vi "LV2Lift.vi"(0 "VerticleMotorControlDevRef":T4={"DeviceStatus"={"status"=FALSE, "code"=0, "source"=""}, "Type"=enum."CAN", "PWM"={"PWM Channel"=enum."PWM 1", "DeadBand"={"Name"="", "maxPositivePwm"=0, "minPositivePwm"=0, "centerPwm"=0, "maxNegativePwm"=0, "minNegativePwm"=0, "angularRange"=0}}, "CAN"={"Device Number"=6, "SetOutput VI Ref"=variant(refnum<vi> refnum), "GetOutput VI Ref"=variant(refnum<vi> refnum), "Enable VI Ref"=variant(refnum<vi> refnum), "Disable VI Ref"=variant(refnum<vi> refnum), "Data"=variant(cluster{"Library":path, "handle":u64, "Control Mode":u16, "UsageFrame":u32, "RefNumName":string, "arbID":u32} {"Library"=path "libCTRE_PhoenixCCI.so", "handle"=53501864, "Control Mode"=0, "UsageFrame"=0, "RefNumName"="LiftElevation", "arbID"=33816582})}, "Invert"=FALSE, "DIO PWM"={"PWM \"Enable\" Channel"=enum."Invalid", "DIOChannel"=enum."Invalid", "PWM Rate"=0.0}}, 9 "Brake DevRef":T1={"DeviceStatus"={"status"=FALSE, "code"=0, "source"=""}, "PWM Channel"=enum."PWM 1", "DeadBand"={"Name"="Servo", "maxPositivePwm"=1770, "minPositivePwm"=1013, "centerPwm"=1007, "maxNegativePwm"=1000, "minNegativePwm"=243, "angularRange"=180}}, 11 "RotationMotorControlDevRef":T4={"DeviceStatus"={"status"=FALSE, "code"=0, "source"=""}, "Type"=enum."CAN", "PWM"={"PWM Channel"=enum."PWM 1", "DeadBand"={"Name"="", "maxPositivePwm"=0, "minPositivePwm"=0, "centerPwm"=0, "maxNegativePwm"=0, "minNegativePwm"=0, "angularRange"=0}}, "CAN"={"Device Number"=7, "SetOutput VI Ref"=variant(refnum<vi> refnum), "GetOutput VI Ref"=variant(refnum<vi> refnum), "Enable VI Ref"=variant(refnum<vi> refnum), "Disable VI Ref"=variant(refnum<vi> refnum), "Data"=variant(cluster{"Library":path, "handle":u64, "Control Mode":u16, "UsageFrame":u32, "RefNumName":string, "arbID":u32} {"Library"=path "libCTRE_PhoenixCCI.so", "handle"=51718392, "Control Mode"=0, "UsageFrame"=0, "RefNumName"="LiftRotation", "arbID"=33816583})}, "Invert"=FALSE, "DIO PWM"={"PWM \"Enable\" Channel"=enum."Invalid", "DIOChannel"=enum."Invalid", "PWM Rate"=0.0}}) -> ()   [LabVIEW 2017]
uses:
  <vilib>/platform/TimedLoop/XDataNode/XDataNode.xnode
  <vilib>/Platform/TimedLoop/XDataNode/nitl_modes.ctl
  <vilib>/Platform/TimedLoop/XDataNode/XDNodeRunTimeDep.lvlib
  <vilib>/Platform/TimedLoop/XDataNode/wakeup.ctl
  <vilib>/Platform/TimedLoop/XDataNode/timing_clust.ctl
  <vilib>/addons/control/pid/NI_PID_pid.lvlib
  <vilib>/addons/control/pid/pid.llb/PID (DBL).vi
  LevelOne/LiftRotLV1Enum.ctl
  LevelOne/VerticalEnum.ctl
  CommandTypes/LiftCommands.ctl
  <vilib>/Rock Robotics/WPI/ThirdParty/Phoenix-LabVIEW/Motor Controller/Controls/CTRE_Phoenix_MotorControl_ControlMode.ctl
  <vilib>/addons/control/pid/pid.llb/PID Output Rate Limiter (DBL).vi
  <vilib>/Rock Robotics/SystemInterfaces/DIO/FPGA_DIOPWMChannel.ctl
  <vilib>/Rock Robotics/WPI/PWM/WPI_PWMDeadband.ctl
  <vilib>/Rock Robotics/WPI/MotorControl/WPI_MotorControlType.ctl
  <vilib>/Rock Robotics/SystemInterfaces/DIO/FPGA_DIOChannel.ctl
  <vilib>/Rock Robotics/WPI/MotorControl/WPI_MotorControlDeviceRef.ctl
  <vilib>/Rock Robotics/WPI/PWM/Servo/WPI_ServoDeviceRef.ctl
panel:
  out "Vertical Lim":cluster{"At Hi":bool, "At Lo":bool}
  out "Vertical Near Lim":cluster{"At Hi near":bool, "At Lo near":bool}
  out "Rotation Arm Current":dbl(graph)
  out "Max Rotation Current":dbl=40.75
  in  "Reset Current Max":bool
  out "Rotation Arm Current":dbl
  in  "Tab Control":T7(tab)=enum."PID"
  in  "Home Desired Rotation":dbl=90.0
  in  "Home Desired Height":dbl=2468.9
  in  "To Scale Low_Desired_Rotation":dbl=54.2584
  in  "To Scale Low_Desired_Height":dbl=16306.2
  in  "To Scale High_Desired_Rotation":dbl=54.2584
  in  "To Scale High_Desired_Height":dbl=26267.9
  in  "To Scale Medium_Desired_Rotation":dbl=54.2584
  in  "To Scale Medium_Desired_Height":dbl=21933.0
  in  "To Switch_Desired_Rotation":dbl=31.0048
  in  "To Switch_Desired_Height":dbl=7119.62
  in  "Ground_Desired_Rotation":dbl
  in  "Ground_Desired_Height":dbl
  in  "Verticle_High_Near_Limit":dbl=4000.0
  in  "Verticle_Low_Limit":dbl=200.0
  in  "Verticle_Low_Near_Limit":dbl=3000.0
  in  "Verticle_Low_Speed_Near_Limit":dbl=0.2
  in  "Verticle_High_Speed_Near_Limit":dbl=0.2
  in  "Verticle_High_Limit":dbl=27000.0
  in  "Vertical coerce":dbl=0.75 format="%#_13g"
  in  "Lift correltion":bool=TRUE
  out "Rotation Tuning Mode?":bool
  in  "Rotation Setpoint":dbl(slide) scale=0.0..100.0
  out "Vertical Tuning Mode?":bool
  in  "Vertical Setpoint":dbl(slide) scale=0.0..30000.0
  out "Vertical Response":cluster{"Value":dbl, "Double":dbl}(graph)={"Value"=7119.62, "Double"=4112.0}
  out "Rotation Response":cluster{"Rotation Setpoint":dbl, "Double":dbl}(graph)={"Rotation Setpoint"=31.0048, "Double"=-8.648384665801359}
  in  "Vertical Min":dbl=-0.9
  in  "Vertical Max":dbl=0.9
  in  "Vertical D Gain":dbl
  in  "Vertical I Gain":dbl
  in  "Vertical P Gain":dbl=0.0001
  in  "Rotation Min":dbl=-1.0
  in  "Rotation Max":dbl=1.0
  in  "Rotation D Gain":dbl=0.002
  in  "Rotation I Gain":dbl=0.01
  in  "Rotation P Gain":dbl=0.03
  in  "rotationalTolerance":dbl=5.0
  in  "Lift_Tolerance":dbl
  in  "Brake Engage Time (s)":dbl
  in  "Brake Servo Engage Angle":dbl
  in  "Brake Servo Disengage Angle":dbl=0.2
  in  "Free_Rotate_Height":dbl=99999.0
  in  "Rotation Feed Forward":dbl(knob)=-0.12604134075051898 scale=1.0..-1.0
  in  "Rot SP Limit":dbl=2000.0 format="%.2f"
  in  "Rotational Manual Power":dbl(knob) scale=0.0..1.0
  in  "Verticle Manual Power":dbl(knob) scale=0.0..1.0
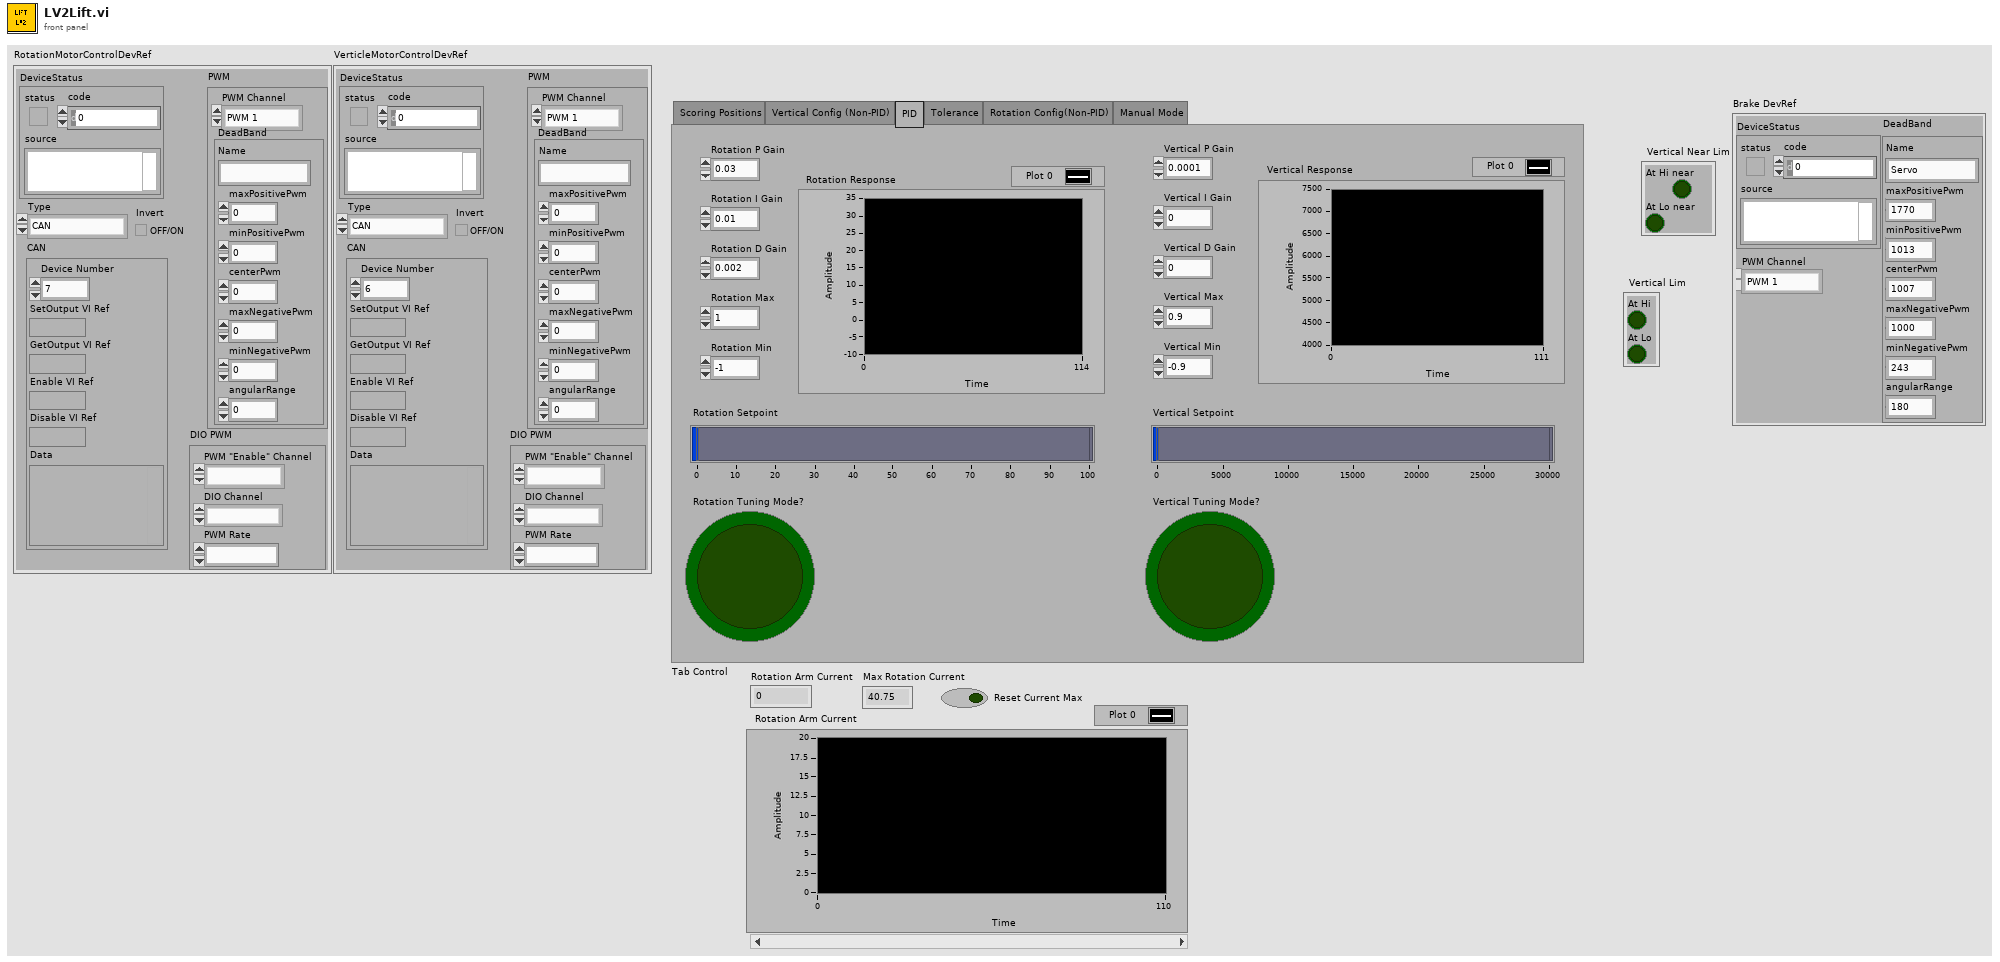
[diagram p1: front panel]
types:
  T1 = typedef "WPI_ServoDeviceRef.ctl" = cluster{"DeviceStatus":errorcluster, "PWM Channel":T2, "DeadBand":T3}
  T2 = typedef "FPGA_DIOPWMChannel.ctl" = enum8{"PWM 0", "PWM 1", "PWM 2", "PWM 3", "PWM 4", "PWM 5", "PWM 6", "PWM 7", "PWM 8", "PWM 9", "PWM MXP 0", "PWM MXP 1", "PWM MXP 2", "PWM MXP 3", "PWM MXP 4", "PWM MXP 5", "PWM MXP 6", "PWM MXP 7", "PWM MXP 8", "PWM MXP 9", "Invalid"}
  T3 = typedef "WPI_PWMDeadband.ctl" = cluster{"Name":string, "maxPositivePwm":i32, "minPositivePwm":i32, "centerPwm":i32, "maxNegativePwm":i32, "minNegativePwm":i32, "angularRange":u16}
  T4 = typedef "WPI_MotorControlDeviceRef.ctl" = cluster{"DeviceStatus":errorcluster, "Type":T5, "PWM":cluster{"PWM Channel":T2, "DeadBand":T3}, "CAN":cluster{"Device Number":u8, "SetOutput VI Ref":variant, "GetOutput VI Ref":variant, "Enable VI Ref":variant, "Disable VI Ref":variant, "Data":variant}, "Invert":bool, "DIO PWM":cluster{"PWM \"Enable\" Channel":T2, "DIOChannel":T6, "PWM Rate":dbl}}
  T5 = typedef "WPI_MotorControlType.ctl" = enum16{"PWM", "CAN", "DIO PWM"}
  T6 = typedef "FPGA_DIOChannel.ctl" = enum8{"DIO 0", "DIO 1", "DIO 2", "DIO 3", "DIO 4", "DIO 5", "DIO 6", "DIO 7", "DIO 8", "DIO 9", "DIO MXP 0", "DIO MXP 1", "DIO MXP 2", "DIO MXP 3", "DIO MXP 4", "DIO MXP 5", "DIO MXP 6", "DIO MXP 7", "DIO MXP 8", "DIO MXP 9", "DIO MXP 10", "DIO MXP 11", "DIO MXP 12", "DIO MXP 13", "DIO MXP 14", "DIO MXP 15", "SPI Port CS1", "SPI Port CS2", "SPI Port CS3", "SPI Port MISO", "SPI Port MOSI", "Invalid"}
  T7 = enum32{"Scoring Positions", "Vertical Config (Non-PID)", "PID", "Tolerance", "Rotation Config(Non-PID)", "Manual Mode"}
  T8 = typedef "LiftCommands.ctl" = enum16{"Do  Nothing", "Manuel", "Home", "Ground", "To Switch", "To Scale Low", "To Scale Medium", "To Scale High"}
  T9 = typedef "XDNodeRunTimeDep.lvlib/timing_clust.ctl" = cluster{"Expected End [f-1]":u64, "Actual End [f-1]":u64, "Finished Late? [f-1]":bool, "Expected End [i-1]":u64, "Actual End [i-1]":u64, "Finished Late? [i-1]":bool, "Expected Start [i]":u64, "Actual Start [i]":u64, "Expected Start [f]":u64, "Actual Start [f]":u64, "Source Name":string, "Structure Name":string, "Period":i64, "Deadline":i64, "Offset":i64, "Start":i64, "Priority":i32, "Timeout":i32, "Mode":T10, "Wakeup Reason":T11, "Error":errorcluster, "Source Type":string, "Secondary Source Type":string, "Global End Time":u64, "Global Start Time":u64, "Frame Duration":u64, "Iteration Duration":u64, "Assigned CPU":i32, "I/O Scan Engine Mode":u32}
  T10 = typedef "XDNodeRunTimeDep.lvlib/nitl_modes.ctl" = enum32{"No Change", "Process missed periods, maintain original phase", "Discard missed periods, maintain original phase", "Process missed periods, ignore original phase", "Discard missed periods, ignore original phase"}
  T11 = typedef "XDNodeRunTimeDep.lvlib/wakeup.ctl" = enum32{"Normal", "Aborted", "Asynchronous wakeup", "Timing source error", "Timed loop error", "Timeout"}
  T12 = typedef "VerticalEnum.ctl" = enum16{"Do Nothing", "Down", "Up"}
  T13 = typedef "LiftRotLV1Enum.ctl" = enum16{"Nothing", "Down", "Up"}
  T14 = cluster{"proportional gain (Kc)":dbl, "integral time (Ti, min)":dbl, "derivative time (Td, min)":dbl}
  T15 = cluster{"Hi Speed near Limit ":dbl, "Lo Speed near Limit":dbl}
  T16 = cluster{"Hi Near Limit ":dbl, "Lo Near Limit":dbl}
  T17 = enum16{"Do  Nothing", "Manuel", "Home", "Ground", "To Switch", "To Scale Low", "To Scale Medium", "To Scale High"}
  T18 = typedef "CTRE_Phoenix_MotorControl_ControlMode.ctl" = u16
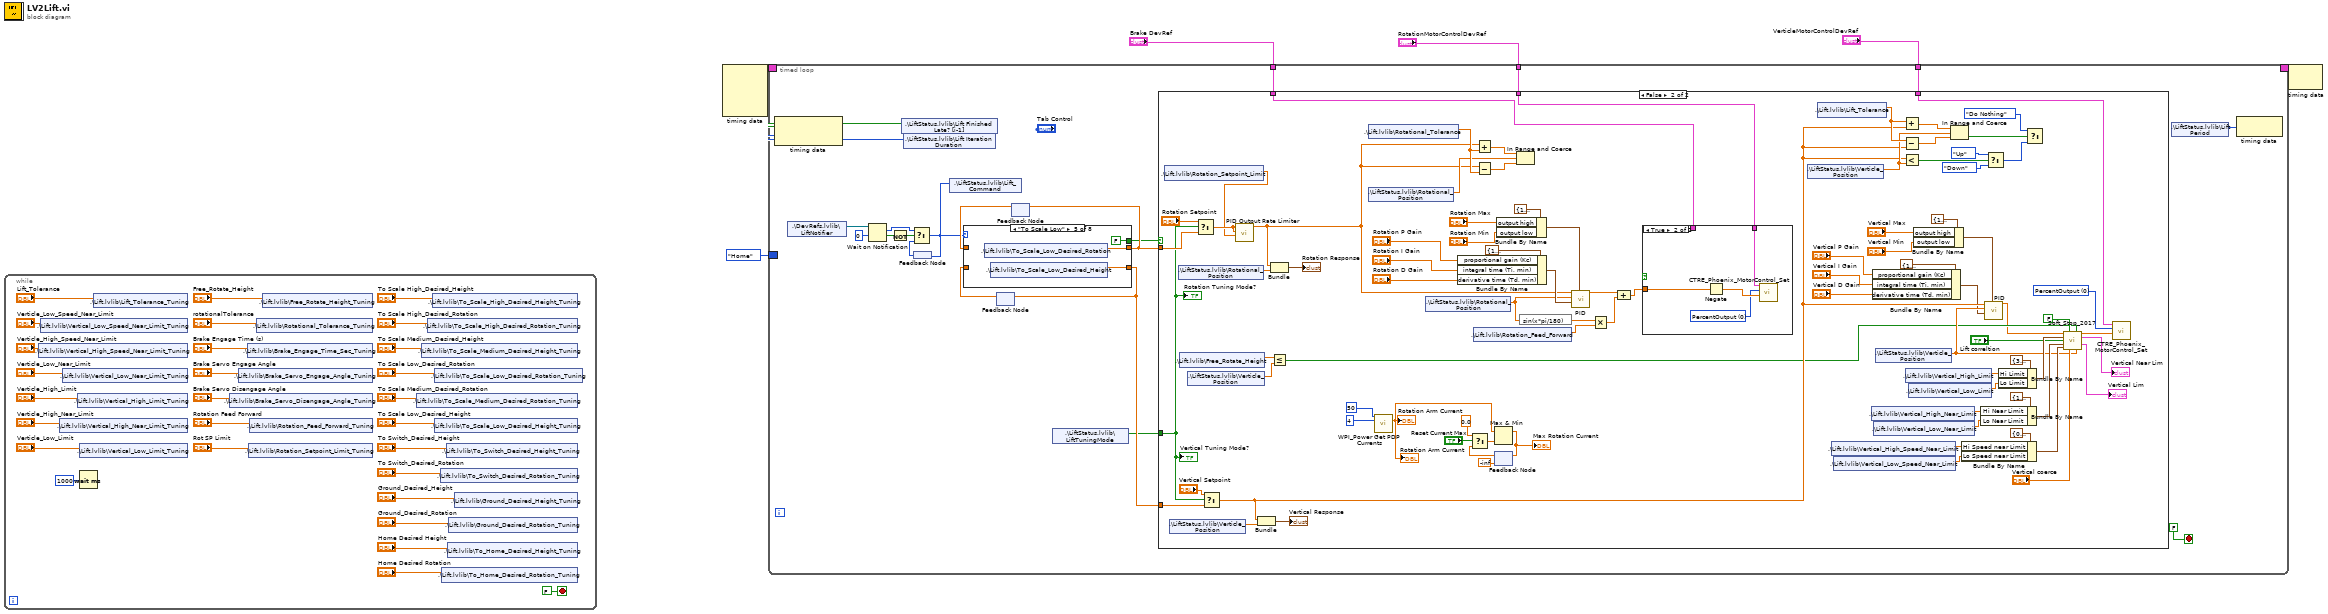
[diagram p0: block diagram]
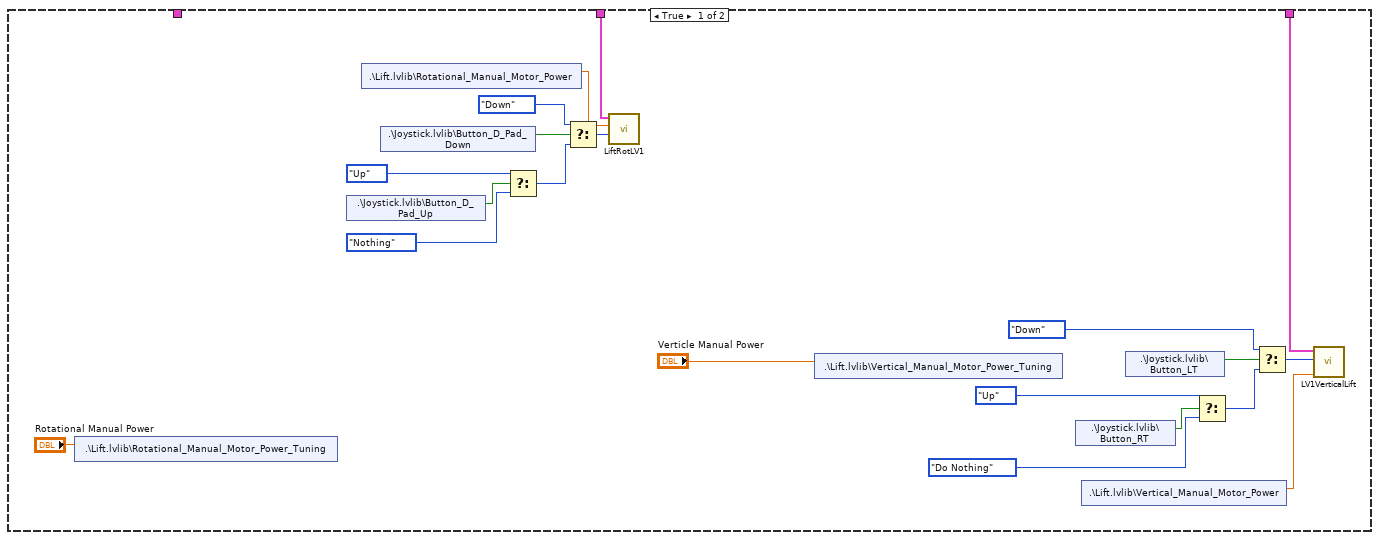
[diagram p2: hidden frame]
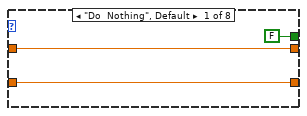
[diagram p4: hidden frame]
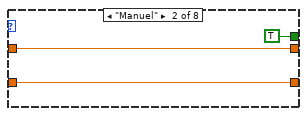
[diagram p5: hidden frame]
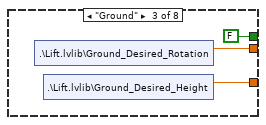
[diagram p6: hidden frame]
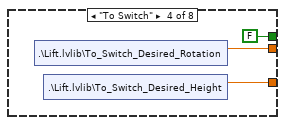
[diagram p7: hidden frame]
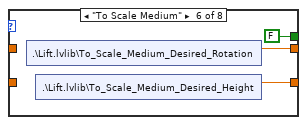
[diagram p8: hidden frame]
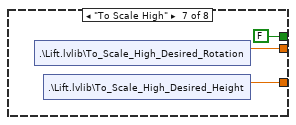
[diagram p9: hidden frame]
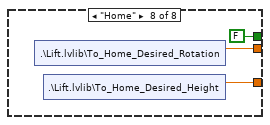
[diagram p10: hidden frame]
diagram:
  n1 = while {
    stop <- FALSE stop-if-true
    n2 = shared-variable ".\\Lift.lvlib\\Vertical_High_Speed_Near_Limit_Tuning"("Verticle_High_Speed_Near_Limit") -> ()  [unwired: 1 in, 1 out]
    n3 = shared-variable ".\\Lift.lvlib\\Vertical_Low_Speed_Near_Limit_Tuning"("Verticle_Low_Speed_Near_Limit") -> ()  [unwired: 1 in, 1 out]
    n4 = shared-variable ".\\Lift.lvlib\\Vertical_High_Near_Limit_Tuning"("Verticle_High_Near_Limit") -> ()  [unwired: 1 in, 1 out]
    n5 = shared-variable ".\\Lift.lvlib\\Vertical_Low_Near_Limit_Tuning"("Verticle_Low_Near_Limit") -> ()  [unwired: 1 in, 1 out]
    n6 = shared-variable ".\\Lift.lvlib\\Vertical_High_Limit_Tuning"("Verticle_High_Limit") -> ()  [unwired: 1 in, 1 out]
    n7 = shared-variable ".\\Lift.lvlib\\Vertical_Low_Limit_Tuning"("Verticle_Low_Limit") -> ()  [unwired: 1 in, 1 out]
    n8 = Wait (ms)(milliseconds to wait=u32 1000) -> ()  [unwired: 1 out]
    n9 = shared-variable ".\\Lift.lvlib\\Lift_Tolerance_Tuning"("Lift_Tolerance") -> ()  [unwired: 1 in, 1 out]
    n10 = shared-variable ".\\Lift.lvlib\\Brake_Servo_Disengage_Angle_Tuning"("Brake Servo Disengage Angle") -> ()  [unwired: 1 in, 1 out]
    n11 = shared-variable ".\\Lift.lvlib\\Brake_Servo_Engage_Angle_Tuning"("Brake Servo Engage Angle") -> ()  [unwired: 1 in, 1 out]
    n12 = shared-variable ".\\Lift.lvlib\\Brake_Engage_Time_Sec_Tuning"("Brake Engage Time (s)") -> ()  [unwired: 1 in, 1 out]
    n13 = shared-variable ".\\Lift.lvlib\\Rotation_Setpoint_Limit_Tuning"("Rot SP Limit") -> ()  [unwired: 1 in, 1 out]
    n14 = shared-variable ".\\Lift.lvlib\\Rotation_Feed_Forward_Tuning"("Rotation Feed Forward") -> ()  [unwired: 1 in, 1 out]
    n15 = shared-variable ".\\Lift.lvlib\\Rotational_Tolerance_Tuning"("rotationalTolerance") -> ()  [unwired: 1 in, 1 out]
    n16 = shared-variable ".\\Lift.lvlib\\Free_Rotate_Height_Tuning"("Free_Rotate_Height") -> ()  [unwired: 1 in, 1 out]
    n17 = shared-variable ".\\Lift.lvlib\\To_Scale_Medium_Desired_Rotation_Tuning"("To Scale Medium_Desired_Rotation") -> ()  [unwired: 1 in, 1 out]
    n18 = shared-variable ".\\Lift.lvlib\\To_Scale_Medium_Desired_Height_Tuning"("To Scale Medium_Desired_Height") -> ()  [unwired: 1 in, 1 out]
    n19 = shared-variable ".\\Lift.lvlib\\To_Scale_High_Desired_Rotation_Tuning"("To Scale High_Desired_Rotation") -> ()  [unwired: 1 in, 1 out]
    n20 = shared-variable ".\\Lift.lvlib\\To_Scale_High_Desired_Height_Tuning"("To Scale High_Desired_Height") -> ()  [unwired: 1 in, 1 out]
    n21 = shared-variable ".\\Lift.lvlib\\To_Scale_Low_Desired_Rotation_Tuning"("To Scale Low_Desired_Rotation") -> ()  [unwired: 1 in, 1 out]
    n22 = shared-variable ".\\Lift.lvlib\\To_Scale_Low_Desired_Height_Tuning"("To Scale Low_Desired_Height") -> ()  [unwired: 1 in, 1 out]
    n23 = shared-variable ".\\Lift.lvlib\\To_Switch_Desired_Rotation_Tuning"("To Switch_Desired_Rotation") -> ()  [unwired: 1 in, 1 out]
    n24 = shared-variable ".\\Lift.lvlib\\To_Home_Desired_Rotation_Tuning"("Home Desired Rotation") -> ()  [unwired: 1 in, 1 out]
    n25 = shared-variable ".\\Lift.lvlib\\To_Switch_Desired_Height_Tuning"("To Switch_Desired_Height") -> ()  [unwired: 1 in, 1 out]
    n26 = shared-variable ".\\Lift.lvlib\\To_Home_Desired_Height_Tuning"("Home Desired Height") -> ()  [unwired: 1 in, 1 out]
    n27 = shared-variable ".\\Lift.lvlib\\Ground_Desired_Rotation_Tuning"("Ground_Desired_Rotation") -> ()  [unwired: 1 in, 1 out]
    n28 = shared-variable ".\\Lift.lvlib\\Ground_Desired_Height_Tuning"("Ground_Desired_Height") -> ()  [unwired: 1 in, 1 out]
  }
  n29 = node-c288() -> (w6:T9)  [unwired: 4 in]
  n30 = timed-loop {
    timing: w6 -> [_]
    timing-out: [_] -> w5
    border: LiftCommands."Home" ("Enum") -> [_]
    tunnel: "VerticleMotorControlDevRef" -> [w43]
    tunnel: "RotationMotorControlDevRef" -> [w42]
    tunnel: "Brake DevRef" -> [w35]
    stop <- FALSE stop-if-true
    n31 = node-c288() -> (w47:bool, w46:i64)  [unwired: 1 in]
    n32 = shared-variable ".\\DevRefs.lvlib\\LiftNotifier"() -> (w54:refnum<notifier>)  [unwired: 1 in, 1 out]
    n33 = Wait on Notification(notifier=w54, timeout in ms (-1)=0) -> (notification=w39:T17, timed out?=w44:bool)  [unwired: 2 in, 2 out]
    n34 = Not(x=w44) -> (.not. x?=w40:bool)
    n35 = shared-variable ".\\LiftStatus.lvlib\\Lift Finished Late? [i-1]"(w47) -> ()  [unwired: 1 in, 1 out]
    n36 = shared-variable ".\\LiftStatus.lvlib\\Lift Iteration Duration"(w46) -> ()  [unwired: 1 in, 1 out]
    n37 = feedback #1() -> (w38:T8)
    n38 = Select(t=w39, s=w40, f=w38) -> (s? t:f=w36:T8)
    n39 = feedback-in #1(w36) -> ()
    n40 = shared-variable ".\\LiftStatus.lvlib\\Lift_Command"(w36) -> ()  [unwired: 1 in, 1 out]
    n41 = feedback #2() -> (w51:dbl)  [unwired: 1 in]
    n42 = feedback #3() -> (w41:dbl)  [unwired: 1 in]
    n43 = case shown="\"To Scale Low\"" w36 {
      tunnel: [w167 w170 w173 w176 w179 w182 w185 w188] -> w50
      tunnel: [w168 w171 w172 w175 w178 w181 w184 w187] -> w52
      tunnel: w51 -> [w168 w171 _ _ _ _ _ _]
      tunnel: w41 -> [w167 w170 _ _ _ _ _ _]
      tunnel: [FALSE TRUE FALSE FALSE FALSE FALSE FALSE FALSE] -> w48
      frame "Do  Nothing", Default {
      }
      frame "Manuel" {
      }
      frame "Ground" {
        n44 = shared-variable ".\\Lift.lvlib\\Ground_Desired_Rotation"() -> (w173:dbl)  [unwired: 1 in, 1 out]
        n45 = shared-variable ".\\Lift.lvlib\\Ground_Desired_Height"() -> (w172:dbl)  [unwired: 1 in, 1 out]
      }
      frame "To Switch" {
        n46 = shared-variable ".\\Lift.lvlib\\To_Switch_Desired_Rotation"() -> (w176:dbl)  [unwired: 1 in, 1 out]
        n47 = shared-variable ".\\Lift.lvlib\\To_Switch_Desired_Height"() -> (w175:dbl)  [unwired: 1 in, 1 out]
      }
      frame "To Scale Low" {
        n48 = shared-variable ".\\Lift.lvlib\\To_Scale_Low_Desired_Rotation"() -> (w179:dbl)  [unwired: 1 in, 1 out]
        n49 = shared-variable ".\\Lift.lvlib\\To_Scale_Low_Desired_Height"() -> (w178:dbl)  [unwired: 1 in, 1 out]
      }
      frame "To Scale Medium" {
        n50 = shared-variable ".\\Lift.lvlib\\To_Scale_Medium_Desired_Rotation"() -> (w182:dbl)  [unwired: 1 in, 1 out]
        n51 = shared-variable ".\\Lift.lvlib\\To_Scale_Medium_Desired_Height"() -> (w181:dbl)  [unwired: 1 in, 1 out]
      }
      frame "To Scale High" {
        n52 = shared-variable ".\\Lift.lvlib\\To_Scale_High_Desired_Rotation"() -> (w185:dbl)  [unwired: 1 in, 1 out]
        n53 = shared-variable ".\\Lift.lvlib\\To_Scale_High_Desired_Height"() -> (w184:dbl)  [unwired: 1 in, 1 out]
      }
      frame "Home" {
        n54 = shared-variable ".\\Lift.lvlib\\To_Home_Desired_Rotation"() -> (w188:dbl)  [unwired: 1 in, 1 out]
        n55 = shared-variable ".\\Lift.lvlib\\To_Home_Desired_Height"() -> (w187:dbl)  [unwired: 1 in, 1 out]
      }
    }
    n56 = feedback-in #2(w52) -> ()
    n57 = feedback-in #3(w50) -> ()
    n58 = shared-variable ".\\LiftStatus.lvlib\\LiftTuningMode"() -> (w37:bool)  [unwired: 1 in, 1 out]
    n59 = case shown="False" w48 {
      tunnel: w52 -> [_ w122]
      tunnel: w50 -> [_ w117]
      tunnel: w43 -> [w59 w82]
      tunnel: w42 -> [w60 w83]
      tunnel: w37 -> [_ w102]
      tunnel: w35 -> [_ w75]
      frame True {
        n60 = shared-variable ".\\Lift.lvlib\\Rotational_Manual_Motor_Power_Tuning"("Rotational Manual Power") -> ()  [unwired: 1 in, 1 out]
        n61 = shared-variable ".\\Joystick.lvlib\\Button_D_Pad_Up"() -> (w66:bool)  [unwired: 1 in, 1 out]
        n62 = shared-variable ".\\Lift.lvlib\\Rotational_Manual_Motor_Power"() -> (w57:dbl)  [unwired: 1 in, 1 out]
        n63 = shared-variable ".\\Joystick.lvlib\\Button_D_Pad_Down"() -> (w65:bool)  [unwired: 1 in, 1 out]
        n64 = Select(t=LiftRotLV1Enum."Up" ("Command"), s=w66, f=LiftRotLV1Enum."Nothing" ("Command")) -> (s? t:f=w74:T13)
        n65 = Select(t=LiftRotLV1Enum."Down" ("Command"), s=w65, f=w74) -> (s? t:f=w72:T13)
        n66 = call "LiftRotLV1.vi"("Command"=w72, "Motor Power"=w57, "PhoenixMotorControlDevRef"=w60) -> ()  [unwired: 9 in]
        n67 = shared-variable ".\\Lift.lvlib\\Vertical_Manual_Motor_Power_Tuning"("Verticle Manual Power") -> ()  [unwired: 1 in, 1 out]
        n68 = shared-variable ".\\Joystick.lvlib\\Button_RT"() -> (w67:bool)  [unwired: 1 in, 1 out]
        n69 = shared-variable ".\\Lift.lvlib\\Vertical_Manual_Motor_Power"() -> (w55:dbl)  [unwired: 1 in, 1 out]
        n70 = shared-variable ".\\Joystick.lvlib\\Button_LT"() -> (w68:bool)  [unwired: 1 in, 1 out]
        n71 = Select(t=VerticalEnum."Up" ("State"), s=w67, f=VerticalEnum."Do Nothing" ("State")) -> (s? t:f=w73:T12)
        n72 = Select(t=VerticalEnum."Down" ("State"), s=w68, f=w73) -> (s? t:f=w61:T12)
        n73 = call "LV1VerticalLift.vi"("Motor Power"=w55, "State"=w61, "PhoenixMotorControlDevRef"=w59) -> ()  [unwired: 9 in]
      }
      frame False {
        w81 = T18 0 items=["PercentOutput"=0, "Position"=1, "Velocity"=2, "Current"=3, "Follower"=5, "MotionProfile"=6, "MotionMagic"=7, "MotionMagicArc"=8, "MotionProfileArc"=10, "Disabled"=15] ("Control Mode")
        n74 = shared-variable ".\\Lift.lvlib\\Rotation_Setpoint_Limit"() -> (w93:dbl)  [unwired: 1 in, 1 out]
        n75 = shared-variable ".\\LiftStatus.lvlib\\Verticle_Position"() -> (w119:dbl)  [unwired: 1 in, 1 out]
        n76 = shared-variable ".\\LiftStatus.lvlib\\Rotational_Position"() -> (w114:dbl)  [unwired: 1 in, 1 out]
        n77 = shared-variable ".\\Lift.lvlib\\Free_Rotate_Height"() -> (w113:dbl)  [unwired: 1 in, 1 out]
        n78 = shared-variable ".\\LiftStatus.lvlib\\Verticle_Position"() -> (w141:dbl)  [unwired: 1 in, 1 out]
        n79 = Select(t="Rotation Setpoint", s=w102, f=w117) -> (s? t:f=w94:dbl)
        n80 = Select(t="Vertical Setpoint", s=w102, f=w122) -> (s? t:f=w120:dbl)
        n81 = call-poly <vilib>:"PID Output Rate Limiter.vi"("output rate (EGU/min)"=w93, "initial output"=w94, "input (controller output)"=w94) -> ("output"=w95:dbl)  [unwired: 5 in, 1 out]
        n82 = Bundle("Double"=w120, "Double"=w119) -> (→"Vertical Response":cluster{"Double":dbl, "Double":dbl})  [unwired: 1 in]
        n83 = Bundle("output"=w95, "Double"=w114) -> (→"Rotation Response":cluster{"output":dbl, "Double":dbl})  [unwired: 1 in]
        n84 = Less Or Equal?(x=w113, y=w141) -> (x <= y?=w101:bool)
        n85 = shared-variable ".\\Lift.lvlib\\Rotational_Tolerance"() -> (w151:dbl)  [unwired: 1 in, 1 out]
        n86 = shared-variable ".\\LiftStatus.lvlib\\Rotational_Position"() -> (w137:dbl)  [unwired: 1 in, 1 out]
        n87 = call <vilib>:"WPI_Power Get PDP Currents.vi"("Power Distribution Panel (0)"=u8 50, "PDP Channel"=4) -> ("current (A)"=w84:dbl)  [unwired: 11 in, 2 out]
        "Rotation Arm Current" <- w84
        "Rotation Arm Current" <- w84
        n88 = shared-variable ".\\LiftStatus.lvlib\\Rotational_Position"() -> (w99:dbl)  [unwired: 1 in, 1 out]
        n89 = Bundle By Name(cluster=T14 {"proportional gain (Kc)"=1.0, "integral time (Ti, min)"=0.01, "derivative time (Td, min)"=0.0} ("PID gains"), "proportional gain (Kc)"="Rotation P Gain", "integral time (Ti, min)"="Rotation I Gain", "derivative time (Td, min)"="Rotation D Gain") -> (w111:T14)
        n90 = shared-variable ".\\Lift.lvlib\\Rotation_Feed_Forward"() -> (w76:dbl)  [unwired: 1 in, 1 out]
        n91 = Add(x=w95, y=w151) -> (x+y=w160:dbl)
        n92 = Subtract(x=w95, y=w151) -> (x-y=w161:dbl)
        n93 = feedback #4(-inf) -> (w89:dbl)
        n94 = Select(t=0.0, s="Reset Current Max", f=w89) -> (s? t:f=w90:dbl)
        n95 = Max & Min(x=w84, y=w90) -> (max(x,y)=w86:dbl)  [unwired: 1 out]
        "Max Rotation Current" <- w86
        n96 = feedback-in #4(w86) -> ()
        n97 = Bundle By Name(cluster=cluster{"output high":dbl, "output low":dbl} {"output high"=100.0, "output low"=-100.0} ("output range"), "output high"="Rotation Max", "output low"="Rotation Min") -> (w112:cluster{"output high":dbl, "output low":dbl})
        n98 = In Range and Coerce(upper limit=w160, x=w137, lower limit=w161) -> ()  [unwired: 2 out]
        n99 = expression code="sin(x*pi/180)"(w99) -> (w98:dbl)
        n100 = call-poly <vilib>:"PID.vi"("output range"=w112, "PID gains"=w111, "process variable"=w99, "setpoint"=w95) -> ("output"=w97:dbl)  [unwired: 6 in, 1 out]
        n101 = Multiply(x=w98, y=w76) -> (x*y=w96:dbl)
        n102 = Compound Arithmetic op=ADD(w97, w96) -> (w77:dbl)
        n103 = case shown="True" {
          selector: _ -> [_ _]
          tunnel: w83 -> [_ w165]
          tunnel: w77 -> [_ w163]
          tunnel: w75 -> [_ _]
          frame False {
          }
          frame True {
            w162 = T18 0 items=["PercentOutput"=0, "Position"=1, "Velocity"=2, "Current"=3, "Follower"=5, "MotionProfile"=6, "MotionMagic"=7, "MotionMagicArc"=8, "MotionProfileArc"=10, "Disabled"=15] ("Control Mode")
            n104 = Negate(x=w163) -> (-x=w164:dbl)
            n105 = call <vilib>:"CTRE_Phoenix_MotorControl_Set.vi"("Output"=w164, "Control Mode"=w162, "PhoenixMotorControlDevRef"=w165) -> ()  [unwired: 7 in, 2 out]
          }
        }
        n106 = shared-variable ".\\LiftStatus.lvlib\\Verticle_Position"() -> (w138:dbl)  [unwired: 1 in, 1 out]
        n107 = shared-variable ".\\Lift.lvlib\\Lift_Tolerance"() -> (w140:dbl)  [unwired: 1 in, 1 out]
        n108 = shared-variable ".\\Lift.lvlib\\Vertical_High_Speed_Near_Limit"() -> (w104:dbl)  [unwired: 1 in, 1 out]
        n109 = shared-variable ".\\Lift.lvlib\\Vertical_Low_Speed_Near_Limit"() -> (w103:dbl)  [unwired: 1 in, 1 out]
        n110 = shared-variable ".\\Lift.lvlib\\Vertical_High_Near_Limit"() -> (w106:dbl)  [unwired: 1 in, 1 out]
        n111 = Bundle By Name(cluster=T14 {"proportional gain (Kc)"=1.0, "integral time (Ti, min)"=0.01, "derivative time (Td, min)"=0.0} ("PID gains"), "proportional gain (Kc)"="Vertical P Gain", "integral time (Ti, min)"="Vertical I Gain", "derivative time (Td, min)"="Vertical D Gain") -> (w109:T14)
        n112 = shared-variable ".\\Lift.lvlib\\Vertical_Low_Near_Limit"() -> (w105:dbl)  [unwired: 1 in, 1 out]
        n113 = shared-variable ".\\LiftStatus.lvlib\\Verticle_Position"() -> (w139:dbl)  [unwired: 1 in, 1 out]
        n114 = Add(x=w140, y=w120) -> (x+y=w157:dbl)
        n115 = Subtract(x=w140, y=w120) -> (x-y=w156:dbl)
        n116 = Less?(x=w120, y=w138) -> (x < y?=w159:bool)
        n117 = shared-variable ".\\Lift.lvlib\\Vertical_High_Limit"() -> (w108:dbl)  [unwired: 1 in, 1 out]
        n118 = shared-variable ".\\Lift.lvlib\\Vertical_Low_Limit"() -> (w107:dbl)  [unwired: 1 in, 1 out]
        n119 = Bundle By Name(cluster=cluster{"output high":dbl, "output low":dbl} {"output high"=100.0, "output low"=-100.0} ("output range"), "output high"="Vertical Max", "output low"="Vertical Min") -> (w110:cluster{"output high":dbl, "output low":dbl})
        n120 = In Range and Coerce(upper limit=w157, x=w138, lower limit=w156) -> (In Range?=w155:bool)  [unwired: 1 out]
        n121 = Bundle By Name(cluster=T15 {"Hi Speed near Limit "=0.04, "Lo Speed near Limit"=0.02} ("Near Speeds"), "Hi Speed near Limit"=w104, "Lo Speed near Limit"=w103) -> (w144:T15)
        n122 = Bundle By Name(cluster=T16 {"Hi Near Limit "=1.0, "Lo Near Limit"=1.0} ("Near Limits"), "Hi Near Limit"=w106, "Lo Near Limit"=w105) -> (w145:T16)
        n123 = call-poly <vilib>:"PID.vi"("output range"=w110, "PID gains"=w109, "process variable"=w139, "setpoint"=w120) -> ("output"=w100:dbl)  [unwired: 6 in, 1 out]
        n124 = Select(t=VerticalEnum."Up" ("State"), s=w159, f=VerticalEnum."Down" ("State")) -> (s? t:f=w152:T12)
        n125 = Bundle By Name(cluster=cluster{"Hi Limit":dbl, "Lo Limit":dbl} {"Hi Limit"=35.0, "Lo Limit"=-10.0} ("Limits"), "Hi Limit"=w108, "Lo Limit"=w107) -> (w148:cluster{"Hi Limit":dbl, "Lo Limit":dbl})
        n126 = Select(t=VerticalEnum."Do Nothing" ("State"), s=w155, f=w152) -> ()  [unwired: 1 out]
        n127 = call <userlib>:"Soft_Stop_2017.vi"("Motor Input"=w100, "Disable Softstops"=FALSE, "Disable Motor"=w101, "Limits"=w148, "correlation"="Lift correltion", "Near Limits"=w145, "Near Speeds"=w144, "motor coerce"="Vertical coerce", "Sense"=w139) -> ("Motor Out"=w78:dbl, "At Near Limits"=→"Vertical Near Lim":cluster{"At Hi near":bool, "At Lo near":bool}, "At limit"=→"Vertical Lim":cluster{"At Hi":bool, "At Lo":bool})  [unwired: 4 in]
        n128 = call <vilib>:"CTRE_Phoenix_MotorControl_Set.vi"("Output"=w78, "Control Mode"=w81, "PhoenixMotorControlDevRef"=w82) -> ()  [unwired: 7 in, 2 out]
        "Vertical Tuning Mode?" <- w102
        "Rotation Tuning Mode?" <- w102
      }
    }
    n129 = shared-variable ".\\LiftStatus.lvlib\\Lift Period"() -> (w45:i64)  [unwired: 1 in, 1 out]
    n130 = node-c288(w45) -> ()  [unwired: 1 out]
  }
  n131 = node-c288(w5) -> ()  [unwired: 1 out]
